vi "LOG_CheckFileSize.vi"(8 "error in (no error)":errorcluster, 10 "maxfilesize":i16, 11 "File":path) -> (0 "error out":errorcluster, 2 "file moved":bool)   [LabVIEW 2016]
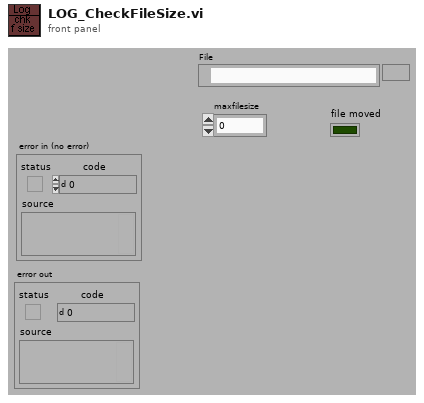
[diagram p1: front panel]
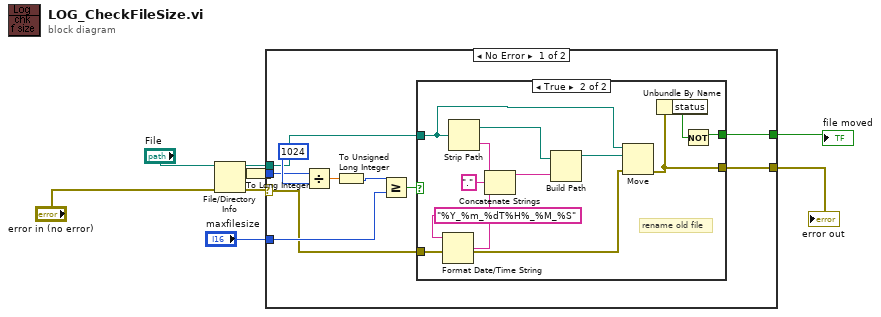
[diagram p0: block diagram]
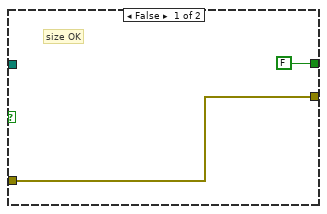
[diagram p2: hidden frame]
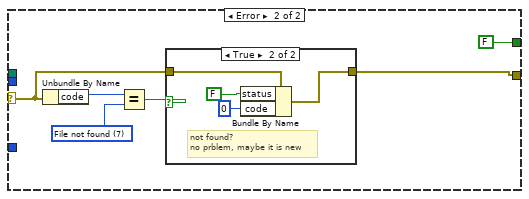
[diagram p3: hidden frame]
diagram:
  n1 = File/Directory Info(path="File", error in="error in (no error)") -> (path out=w5:path, size=w1:i64, error out=w4:errorcluster)  [unwired: 4 out]
  n2 = To Long Integer(number=w1) -> (32bit integer=w7:i32)
  n3 = case shown="No Error" w4 {
    selector: w4 -> [w11 w35]
    tunnel: "maxfilesize" -> [w19 _]
    tunnel: w7 -> [w16 _]
    tunnel: w5 -> [w14 _]
    tunnel: [w12 w34] -> w3
    tunnel: [w10 FALSE ("f")] -> w2
    frame No Error {
      n4 = Divide(x=w16, y=1024) -> (x/y=w17:dbl)
      n5 = To Unsigned Long Integer(number=w17) -> (unsigned 32bit integer=w15:u32)
      n6 = Greater Or Equal?(x=w15, y=w19) -> (x >= y?=w13:bool)
      n7 = case shown="True" w13 {
        tunnel: w14 -> [_ w26]
        tunnel: [w21 w24] -> w12
        tunnel: w11 -> [w21 w27]
        tunnel: [FALSE ("f") w22] -> w10
        frame False {
          # "size OK"
        }
        frame True {
          # "rename old file"
          n8 = Format Date/Time String(time format string (%c)="%Y_%m_%dT%H%_%M_%S") -> (date/time string=w30:string)  [unwired: 2 out]
          n9 = Strip Path(path=w26) -> (stripped path=w25:path, name=w33:string)
          n10 = Concatenate Strings(w33, "." ("string"), w30) -> (w29:string)
          n11 = Build Path(base path=w25, name or relative path=w29) -> (appended path=w28:path)
          n12 = Move(source path=w26, error in=w27, 10:w28) -> (error out=w24:errorcluster)  [unwired: 4 out]
          n13 = Unbundle By Name(w24) -> ("status"=w23:bool)
          n14 = Not(x=w23) -> (.not. x?=w22:bool)
        }
      }
    }
    frame Error {
      w37 = 7 items=["No error", "Argument error", "Memory is full", "Out of zone", "End of file", "File already open", "Generic file I/O error", "File not found", "File permission error", "Disk is full", "Duplicate path", "Too many files open", "System feature not enabled", "Resource file not found", "Cannot add resource", "Resource not found", "Image not found", "Image memory error", "Pen does not exist", "Config type invalid", "Config token not found", "Config parse error", "Config memory error", "Bad external code format", "Bad external code offset", "External code not present", "Null window", "Destroy window error", "Null menu", "Print aborted", "Bad print record", "Print driver error", "Windows error during printing", "Memory error during printing", "Print dialog error", "Generic print error", "Invalid device refnum", "Device not found", "Device parameter error", "Device unit error", "Cannot open device", "Device call aborted", "Generic error", "Cancelled by user", "Object ID too low", "Object ID too high", "Object not in heap", "Unknown heap", "Unknown object (invalid DefProc)", "Unknown object (DefProc not in table)", "Message out of range", "Invalid (null) method", "Unknown message", "Manager call not supported", "Bad address", "Network operation in progress", "Network operation timed out", "Connection is busy", "Network attribute not supported", "Network error", "Address in use", "System out of memory", "Connection aborted", "Connection refused", "Not connected", "Already connected", "Connection closed", "Initialization error (interapplication manager)", "Bad occurrence", "Wait on unbound occurrence handler", "Occurrence queue overflow", "Datalog type conflict", "Unused", "Unrecognized type (interapplication manager)", "Memory corrupt", "Failed to make temporary DLL", "Old CIN version", "Drag socket not found", "Failed to load drop-object", "Failed to register OLE object", "Failed to release OLE object", "Format specifier type mismatch", "Unknown format specifier", "Too few format specifiers", "Too many format specifiers", "Scan failed", "Newer CIN version", "Error converting to variant", "Runtime menu error", "Password tampered", "Variant attribute not found", "Incompatible variant data type", "Event data is not available", "Event Store is not present", "Occurrence is not found", "Event Queue is not created", "Event info is not available", "Refnum passed is NULL", "Error retrieving Class GUID", "Error retrieving CoClass GUID", "Error retrieving TypeLib GUID.", "Bad built application magic bytes.", "Specific driver is different from the specific driver associated with the Logical Name.", "There is no session opened to the class driver.", "Max Error", "MAX - Error with config objects", "MAX - Error loading configuration", "MAX - Group not supported"]
      n15 = Unbundle By Name(w35) -> ("code"=w38:i32)
      n16 = Equal?(x=w38, y=w37) -> (x = y?=w36:bool)
      n17 = case shown="True" w36 {
        tunnel: w35 -> [w40 w44]
        tunnel: [w40 w41] -> w34
        frame False {
        }
        frame True {
          # "not found?\nno prblem, maybe it is new"
          n18 = Bundle By Name(cluster=w44, "status"=FALSE, "code"=0) -> (w41:errorcluster)
        }
      }
    }
  }
  "error out" <- w3
  "file moved" <- w2
